vi "qn_Inverse Hessian update.vi"(7 "reset":bool, 8 "zeta":dbl=1.0, 9 "gradient":dbl[](array[numeric]), 10 "X":dbl[](array[numeric])) -> (0 "error out":errorcluster, 3 "Dk+1":dbl[][](array[numeric]))   [LabVIEW 2017, in "NI_Gmath.lvlib"]
uses:
  <vilib>/gmath/NI_Gmath.lvlib
  <vilib>/Analysis/baseanly.llb/Real Outer Product.vi
  <vilib>/Analysis/baseanly.llb/Real Dot Product.vi
  <vilib>/Analysis/baseanly.llb/A x Vector.vi
  <vilib>/Analysis/baseanly.llb/Real A x B.vi
  <vilib>/Analysis/Matrix/Numeric/Conversions/Matrix To Array - RM.vi
  <vilib>/Analysis/7linalg.llb/Create Special Real Matrix.vi
  <vilib>/Analysis/Matrix/Numeric/Conversions/Array To Matrix - RA2.vi
  <vilib>/Analysis/Matrix/Numeric/Multiply/Multiply - RM,R.vi
  <vilib>/Analysis/NI_AALBase.lvlib
  <vilib>/Analysis/NI_AALPro.lvlib
  <vilib>/Analysis/Matrix/NI_Matrix.lvlib
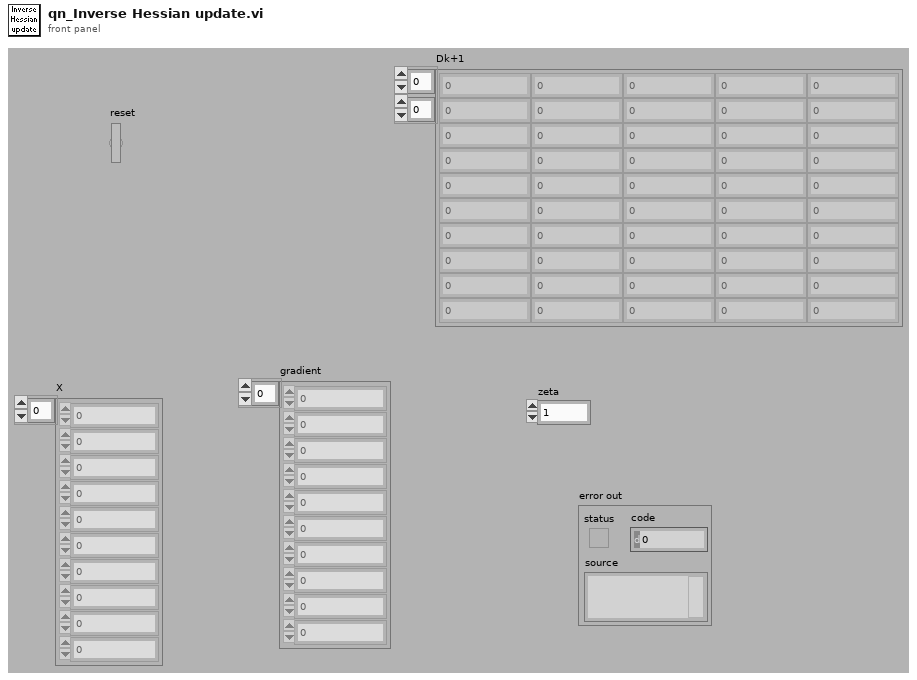
[diagram p1: front panel]
types:
  T1 = enum32{"Identity", "Diagonal", "Toepliz", "Vandermonde", "Companion"}
  T2 = typedef "NI_Matrix.lvlib/RealMatrix.ctl" = dbl[][]
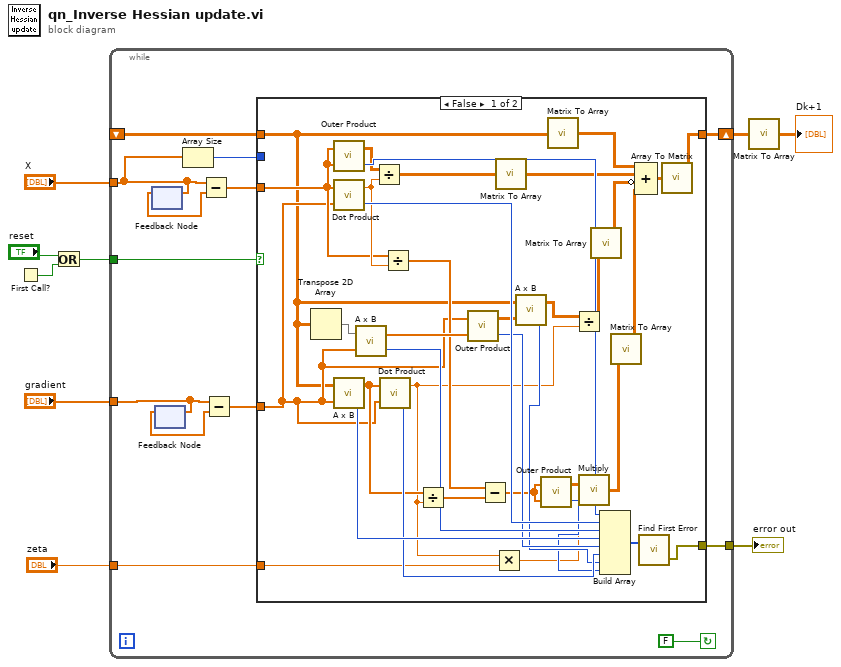
[diagram p0: block diagram]
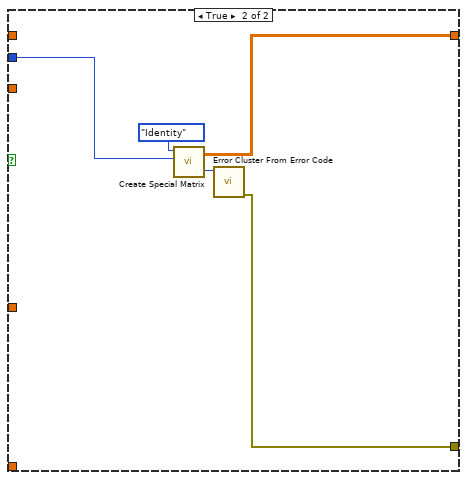
[diagram p2: hidden frame]
diagram:
  n1 = First Call?() -> (First Call?: T/F=w2:bool)
  n2 = Or(x="reset", y=w2) -> (x .or. y?=w1:bool)
  n3 = while {
    tunnel: "X" -> [w12]
    tunnel: "zeta" -> [w22]
    tunnel: "gradient" -> [w17]
    shift-right: [w15] -> w5
    shift-left: _ -> [w14]
    tunnel: w1 -> [w13]
    tunnel: [w10] -> w6
    stop <- FALSE continue-if-true
    n4 = feedback-in #1(w12) -> ()
    n5 = feedback #1() -> (w20:dbl[])  [unwired: 1 in]
    n6 = feedback-in #2(w17) -> ()
    n7 = feedback #2() -> (w18:dbl[])  [unwired: 1 in]
    n8 = Array Size(array=w12) -> (size(s)=w11:i32)
    n9 = Subtract(x=w12, y=w20) -> (x-y=w19:dbl[])
    n10 = Subtract(x=w17, y=w18) -> (x-y=w16:dbl[])
    n11 = case shown="False" w13 {
      tunnel: w22 -> [w37 _]
      tunnel: w19 -> [w33 _]
      tunnel: w16 -> [w32 _]
      tunnel: [w23 w59] -> w15
      tunnel: w14 -> [w24 _]
      tunnel: w11 -> [_ w61]
      tunnel: [w31 w60] -> w10
      frame False {
        n12 = Transpose 2D Array(2D array=w24) -> (transposed array=w48:T2)
        n13 = call-poly <vilib>:"Outer Product.vi"("Y Vector"=w33, "X Vector"=w33) -> ("error"=w58:i32, "Outer Product"=w50:T2)
        n14 = call-poly <vilib>:"Dot Product.vi"("Y Vector"=w32, "X Vector"=w33) -> ("error"=w57:i32, "X * Y"=w42:dbl)
        n15 = call-poly <vilib>:"A x B.vi"("Vector"=w32, "A"=w24) -> ("error"=w55:i32, "A x Vector"=w43:dbl[])
        n16 = call-poly <vilib>:"A x B.vi"("Vector"=w32, "A"=w48) -> ("error"=w56:i32, "A x Vector"=w47:dbl[])
        n17 = Divide(x=w50, y=w42) -> (x/y=w49:T2)
        n18 = call-poly <vilib>:"Dot Product.vi"("Y Vector"=w32, "X Vector"=w43) -> ("error"=w53:i32, "X * Y"=w38:dbl)
        n19 = Divide(x=w33, y=w42) -> (x/y=w41:dbl[])
        n20 = Divide(x=w43, y=w38) -> (x/y=w40:dbl[])
        n21 = call-poly <vilib>:"Outer Product.vi"("Y Vector"=w47, "X Vector"=w32) -> ("error"=w54:i32, "Outer Product"=w46:T2)
        n22 = Subtract(x=w41, y=w40) -> (x-y=w39:dbl[])
        n23 = Multiply(x=w38, y=w37) -> (x*y=w35:dbl)
        n24 = call-poly <vilib>:"Matrix To Array.vi"("Real Matrix"=w49) -> ("Real 2D Array"=w29:dbl[][])
        n25 = call-poly <vilib>:"A x B.vi"("B"=w46, "A"=w24) -> ("error"=w52:i32, "A x B"=w45:T2)
        n26 = call-poly <vilib>:"Outer Product.vi"("Y Vector"=w39, "X Vector"=w39) -> ("error"=w51:i32, "Outer Product"=w36:T2)
        n27 = call-poly <vilib>:"Matrix To Array.vi"("Real Matrix"=w24) -> ("Real 2D Array"=w25:dbl[][])
        n28 = Divide(x=w45, y=w38) -> (x/y=w44:T2)
        n29 = call-poly <vilib>:"Multiply.vi"("Real Scalar c"=w35, "Real Matrix A"=w36) -> ("A * c"=w34:T2)
        n30 = call-poly <vilib>:"Matrix To Array.vi"("Real Matrix"=w44) -> ("Real 2D Array"=w28:dbl[][])
        n31 = Build Array(w58, w57, w56, w55, w54, w53, w52, w51) -> (w30:i32[])
        n32 = call-poly <vilib>:"Matrix To Array.vi"("Real Matrix"=w34) -> ("Real 2D Array"=w27:dbl[][])
        n33 = Compound Arithmetic op=ADD(w25, w29, invert w28, w27) -> (w26:dbl[][])
        n34 = call <vilib>:"Find First Error.vi"("error codes"=w30) -> ("error out"=w31:errorcluster)  [unwired: 3 in, 1 out]
        n35 = call-poly <vilib>:"Array To Matrix.vi"("Real 2D Array"=w26) -> ("Real Matrix"=w23:T2)
      }
      frame True {
        n36 = call-poly <vilib>:"Create Special Matrix.vi"("matrix type"=T1."Identity", "matrix size"=w61) -> ("Special Matrix"=w59:T2, "error"=w63:i32)  [unwired: 3 in]
        n37 = call <vilib>:"Error Cluster From Error Code.vi"("error code (0)"=w63) -> ("error out"=w60:errorcluster)  [unwired: 8 in]
      }
    }
  }
  "error out" <- w6
  n38 = call-poly <vilib>:"Matrix To Array.vi"("Real Matrix"=w5) -> ("Real 2D Array"=→"Dk+1":dbl[][])
